vi "add_batch_ID_pair_to_batch_ID_buffer.vi"(6 "recordset_in":variant[][](array[variant]), 8 "error_in":errorcluster, 10 "BATCH_NUMBER":string, 11 "SQL_batch_ID_buffer_all_info_in":T1) -> (0 "error_out":errorcluster, 1 "BATCH_ID_out":string, 2 "PART_NUMBER exists?":bool, 3 "SQL_batch_ID_buffer_all_info_out":T1)   [LabVIEW 2020]
uses:
  SQL_batch_ID_buffer_all_info.ctl
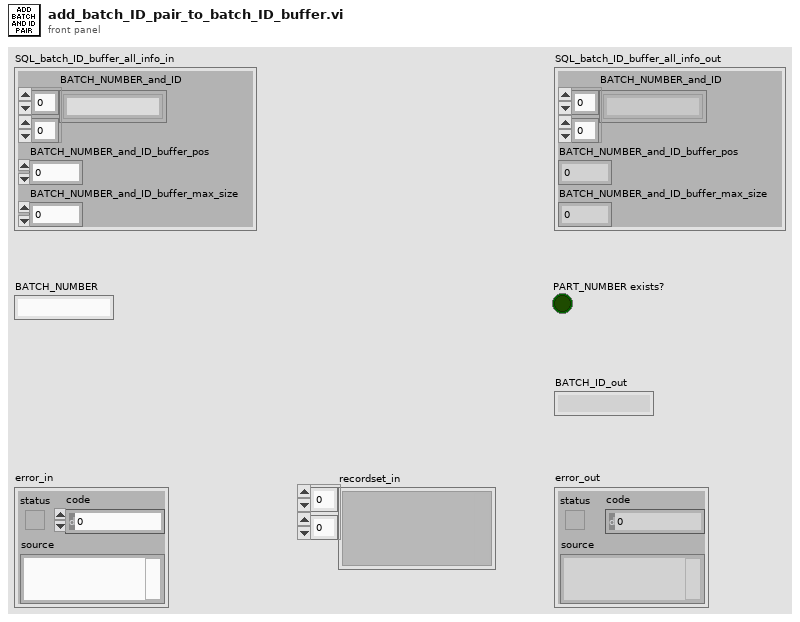
[diagram p1: front panel]
types:
  T1 = typedef "SQL_batch_ID_buffer_all_info.ctl" = cluster{"BATCH_NUMBER_and_ID":string[][], "BATCH_NUMBER_and_ID_buffer_pos":i32, "BATCH_NUMBER_and_ID_buffer_max_size":i32}
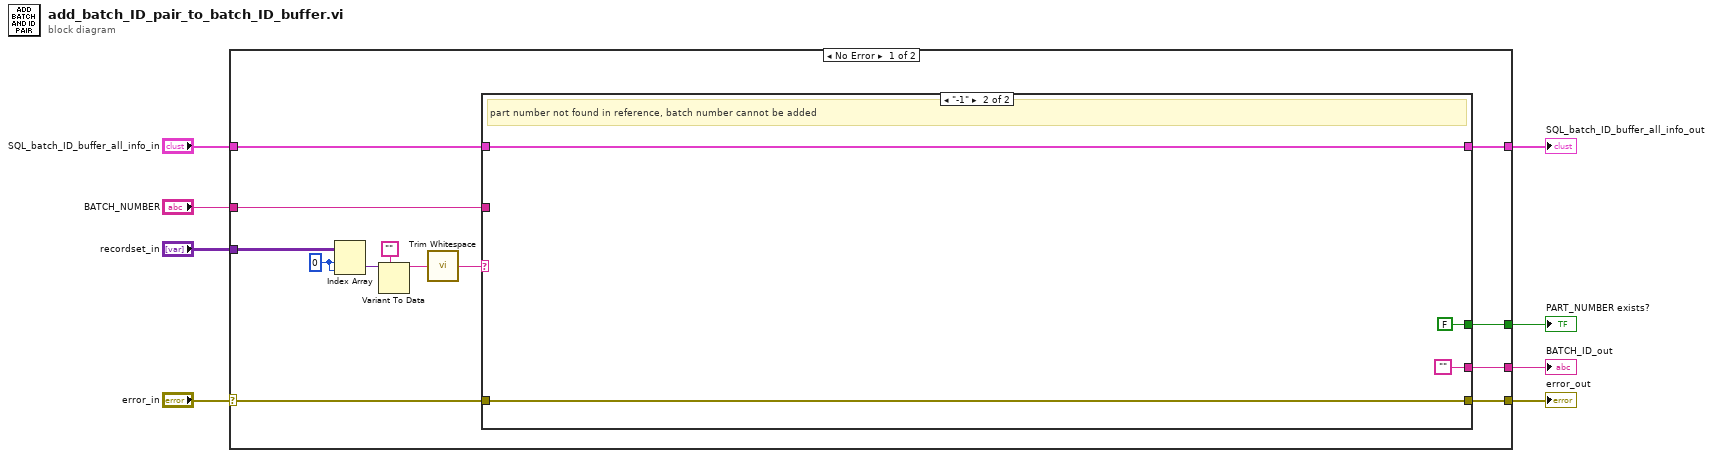
[diagram p0: block diagram]
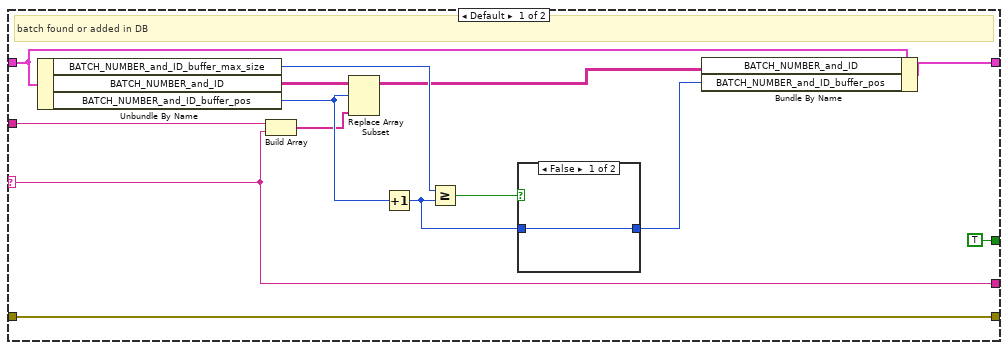
[diagram p2: hidden frame]
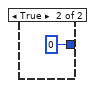
[diagram p3: hidden frame]
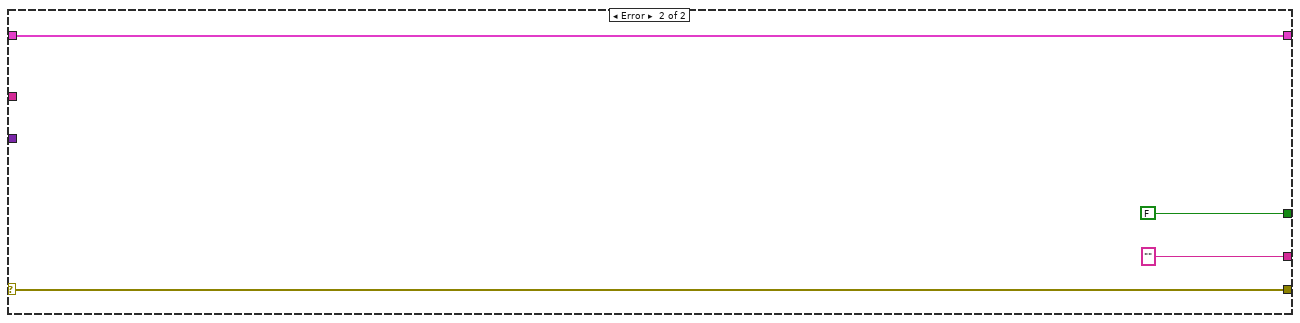
[diagram p4: hidden frame]
diagram:
  n1 = case shown="No Error" "error_in" {
    selector: "error_in" -> [w17 w45]
    tunnel: [w21 w44] -> w8
    tunnel: "SQL_batch_ID_buffer_all_info_in" -> [w20 w44]
    tunnel: "BATCH_NUMBER" -> [w19 _]
    tunnel: [w16 w45] -> w4
    tunnel: "recordset_in" -> [w10 _]
    tunnel: [w18 "" ("trimmed string")] -> w2
    tunnel: [w15 FALSE] -> w1
    frame No Error {
      w11 = 0 ("index")
      n2 = Index Array(array=w10, index (row)=w11, index (col)=w11) -> (element=w12:variant)
      n3 = Variant To Data(type="", Variant=w12) -> (data=w13:string)  [unwired: 1 in, 1 out]
      n4 = call <vilib>:"Trim Whitespace.vi"("string"=w13) -> ("trimmed string"=w9:string)  [unwired: 1 in]
      n5 = case shown="\"-1\"" w9 {
        selector: w9 -> [w22 _]
        tunnel: [w29 w41] -> w21
        tunnel: w20 -> [w28 w41]
        tunnel: w19 -> [w26 _]
        tunnel: [w22 ""] -> w18
        tunnel: w17 -> [w24 w40]
        tunnel: [w24 w40] -> w16
        tunnel: [TRUE FALSE] -> w15
        frame Default {
          # "batch found or added in DB"
          n6 = Unbundle By Name(w28) -> ("BATCH_NUMBER_and_ID_buffer_max_size"=w33:i32, "BATCH_NUMBER_and_ID"=w25:string[][], "BATCH_NUMBER_and_ID_buffer_pos"=w31:i32)
          n7 = Build Array(w26, w22) -> (w27:string[])
          n8 = Replace Array Subset(array=w25, new element=w27, index (row)=w31) -> (w30:string[][])  [unwired: 1 in]
          n9 = Increment(x=w31) -> (x+1=w34:i32)
          n10 = Greater Or Equal?(x=w33, y=w34) -> (x >= y?=w32:bool)
          n11 = case shown="False" w32 {
            tunnel: w34 -> [w36 _]
            tunnel: [w36 0] -> w35
            frame False {
            }
            frame True {
            }
          }
          n12 = Bundle By Name(cluster=w28, "BATCH_NUMBER_and_ID"=w30, "BATCH_NUMBER_and_ID_buffer_pos"=w35) -> (w29:T1)
        }
        frame "-1" {
          # "part number not found in reference, batch number cannot be added"
        }
      }
    }
    frame Error {
    }
  }
  "SQL_batch_ID_buffer_all_info_out" <- w8
  "error_out" <- w4
  "BATCH_ID_out" <- w2
  "PART_NUMBER exists?" <- w1
